vi "MotorPosition.vi"() -> ()   [LabVIEW 2016]
panel:
  out "Request Z-Position":dbl
  out "Z-Position":dbl
  out "Y-Position":dbl
  out "X-Position":dbl
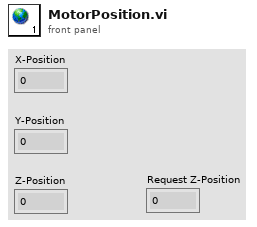
[diagram p1: front panel]
diagram:
